vi "GetListenerProcessList.vi"(8 "error in (no error)":errorcluster, 11 "Qbus in":refnum<class "Qbus.lvclass">) -> (0 "error in (no error)":errorcluster, 1 "processes":string[](array[string]), 3 "Qbus out":refnum<class "Qbus.lvclass">)   [LabVIEW 2017, in "Qbus.lvclass"]
uses:
  <vilib>/addons/Qbus/Qbus.lvclass
  <vilib>/addons/Qbus/Qbus.lvclass/Qbus.ctl
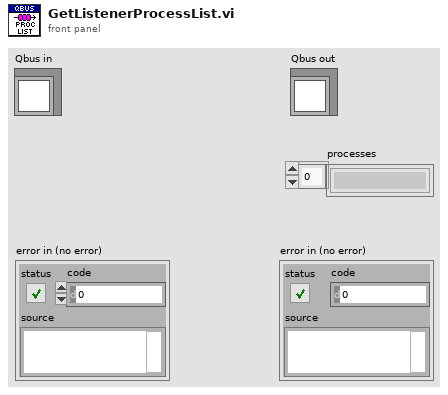
[diagram p1: front panel]
types:
  T1 = typedef "Qbus.lvclass/data.ctl" = cluster{"Queues":variant, "Subscriptions":variant, "MasterQ":string}
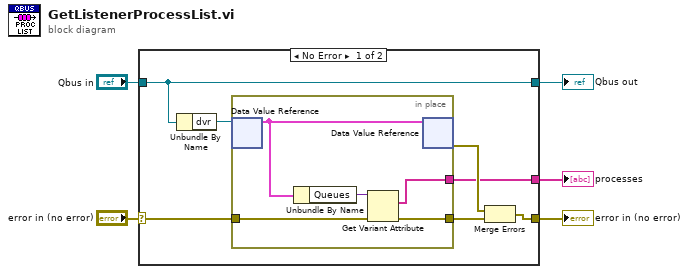
[diagram p0: block diagram]
diagram:
  n1 = case shown="No Error" "error in (no error)" {
    selector: "error in (no error)" -> [w9 w19]
    tunnel: [w8 w19] -> w4
    tunnel: [w12 w18] -> w2
    tunnel: "Qbus in" -> [w12 w18]
    tunnel: [w6 _] -> w1
    frame No Error {
      n2 = Unbundle By Name(w12) -> ("dvr"=w11:refnum<data-value>)
      n3 = in-place {
        in-place-border: w9 -> [w17]
        in-place-border: [w14] -> w7
        in-place-border: [w13] -> w6
        n4 = in-place-dvr #1(w11) -> (w15:T1)  [unwired: 1 out]
        n5 = Unbundle By Name(w15) -> ("Queues"=w16:variant)
        n6 = Get Variant Attribute(Variant=w16, error in=w17) -> (names=w13:string[], error out=w14:errorcluster)  [unwired: 2 in, 2 out]
        n7 = in-place-dvr #1(w15) -> (w10:errorcluster)  [unwired: 1 out]
      }
      n8 = Merge Errors(w10, w7) -> (w8:errorcluster)
    }
    frame Error {
    }
  }
  "error in (no error)" <- w4
  "Qbus out" <- w2
  "processes" <- w1
